vi "Windowing.vi"(6 "Sample rate":i32, 9 "Window length (s)":dbl, 10 "Window overlay (s)":dbl, 11 "x":dbl[](array[numeric])) -> (3 "Windowed array":dbl[][](array[numeric]))   [LabVIEW 2019]
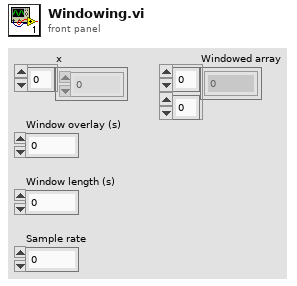
[diagram p1: front panel]
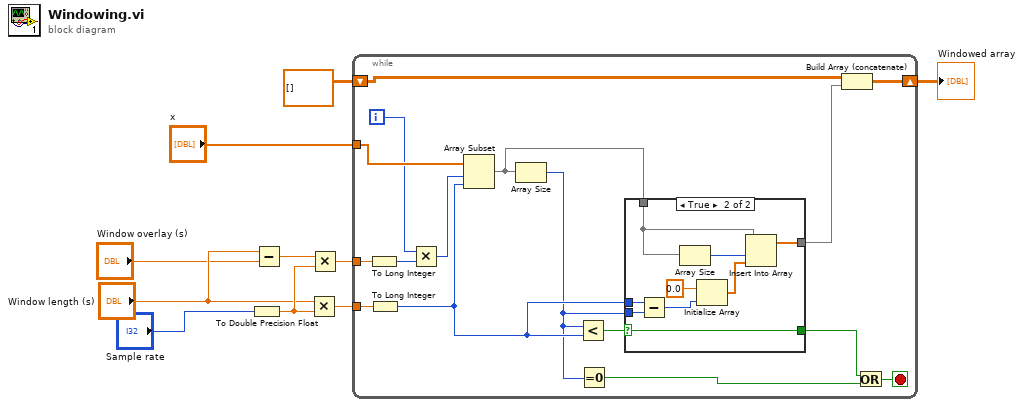
[diagram p0: block diagram]
diagram:
  n1 = To Double Precision Float(number="Sample rate") -> (double precision float=w6:dbl)
  n2 = Subtract(x="Window length (s)", y="Window overlay (s)") -> (x-y=w5:dbl)
  n3 = Multiply(x="Window length (s)", y=w6) -> (x*y=w8:dbl)
  n4 = Multiply(x=w5, y=w6) -> (x*y=w7:dbl)
  n5 = while {
    tunnel: "x" -> [w25]
    tunnel: w8 -> [w26]
    tunnel: w7 -> [w24]
    shift-right: [w13] -> w10
    shift-left: dbl[][] [] -> [w12]
    i -> [w15]
    stop <- w20 stop-if-true
    n6 = To Long Integer(number=w24) -> (32bit integer=w17:i32)
    n7 = To Long Integer(number=w26) -> (32bit integer=w22:i32)
    n8 = Multiply(x=w15, y=w17) -> (x*y=w16:i32)
    n9 = Array Subset(array=w25, index=w16, length=w22) -> (w14:dbl[])
    n10 = Array Size(array=w14) -> (size(s)=w21:i32)
    n11 = Less?(x=w21, y=w22) -> (x < y?=w23:bool)
    n12 = Equal To 0?(x=w21) -> (x = 0?=w18:bool)
    n13 = case shown="True" w23 {
      selector: w23 -> [w27 w29]
      tunnel: w14 -> [w28 w31]
      tunnel: w22 -> [_ w35]
      tunnel: w21 -> [_ w34]
      tunnel: [w28 w32] -> w11
      tunnel: [w27 w29] -> w19
      frame False {
      }
      frame True {
        n14 = Subtract(x=w35, y=w34) -> (x-y=w36:i32)
        n15 = Array Size(array=w31) -> (size(s)=w30:i32)
        n16 = Initialize Array(0.0 ("element"), w36) -> (w33:dbl[])
        n17 = Insert Into Array(array=w31, index=w30, new element=w33) -> (w32:dbl[])
      }
    }
    n18 = Build Array (concatenate)(w12, w11) -> (w13:dbl[][])
    n19 = Or(x=w19, y=w18) -> (x .or. y?=w20:bool)
  }
  "Windowed array" <- w10
